vi "SUB_DELETE_SpecificFile.vi"(3 "Filename to be  Deleted":string) -> (0 "error out":errorcluster)   [LabVIEW 2011]
panel:
  out "File Existing True/Flase":bool
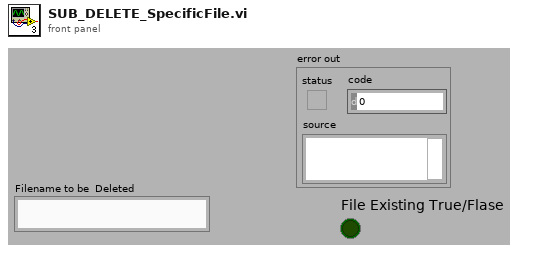
[diagram p1: front panel]
types:
  T1 = enum32{"invalid app kind", "Development System", "Run Time System", "Student Edition", "Embedded LabVIEW", "Evaluation", "Custom"}
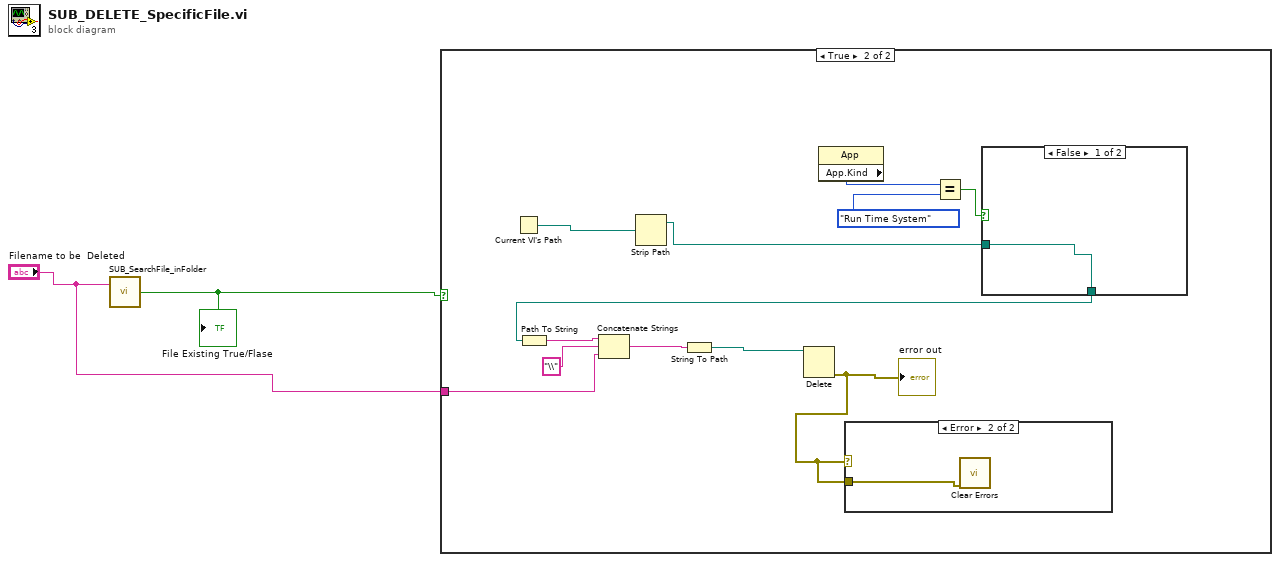
[diagram p0: block diagram]
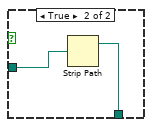
[diagram p4: hidden frame]
diagram:
  n1 = call "SUB_SearchFile_inFolder.vi"("Search Filename in Folder"="Filename to be  Deleted") -> ("File Existing True/Flase"=w2:bool)  [unwired: 1 in]
  "File Existing True/Flase" <- w2
  n2 = case shown="True" w2 {
    tunnel: "Filename to be  Deleted" -> [_ w4]
    frame False {
    }
    frame True {
      n3 = Current VI's Path() -> (path=w14:path)
      n4 = Strip Path(path=w14) -> (stripped path=w10:path)  [unwired: 1 out]
      n5 = property class="App"() -> ("App.Kind"=w13:T1)  [unwired: 2 in, 2 out]
      n6 = Equal?(x=w13, y=T1."Run Time System" ("Application:Kind")) -> (x = y?=w11:bool)
      n7 = case shown="False" w11 {
        tunnel: w10 -> [w16 w18]
        tunnel: [w16 w17] -> w9
        frame False {
        }
        frame True {
          n8 = Strip Path(path=w18) -> (stripped path=w17:path)  [unwired: 1 out]
        }
      }
      n9 = Path To String(path=w9) -> (string=w8:string)
      n10 = Concatenate Strings(w8, "\\" ("string"), w4) -> (w6:string)
      n11 = String To Path(string=w6) -> (path=w5:path)
      n12 = Delete(path (use dialog)=w5) -> (error out=w3:errorcluster)  [unwired: 4 in, 2 out]
      "error out" <- w3
      n13 = case shown="Error" w3 {
        tunnel: w3 -> [_ w15]
        frame No Error {
        }
        frame Error {
          n14 = call <vilib>:"Clear Errors.vi"("error in (no error)"=w15) -> ()  [unwired: 6 in, 1 out]
        }
      }
    }
  }
